vi "flyback scan with VIS monitor.vi"() -> ()   [LabVIEW 2015]
uses:
  <vilib>/DAQmx/read.llb/DAQmx Read (Analog 1D DBL 1Chan NSamp).vi
  <vilib>/DAQmx/write.llb/DAQmx Write (Digital 1D U32 1Chan NSamp).vi
  <vilib>/DAQmx/create/channels.llb/DAQmx Create Channel (DO-Digital Output).vi
  <vilib>/DAQmx/create/channels.llb/DAQmx Create Channel (CO-Pulse Generation-Time).vi
  <vilib>/DAQmx/configure/trigger.llb/DAQmx Start Trigger (Digital Edge).vi
  <vilib>/DAQmx/create/channels.llb/DAQmx Create Channel (AI-Voltage-Basic).vi
  <vilib>/DAQmx/configure/timing.llb/DAQmx Timing (Sample Clock).vi
  <vilib>/DAQmx/miscellaneous.llb/DAQmx Fill In Error Info.vi
  <vilib>/DAQmx/create/channels.llb/DAQmx Create Channel (CO-Pulse Generation-Frequency).vi
  <vilib>/DAQmx/configure/timing.llb/DAQmx Timing (Implicit).vi
  <resource>/objmgr/daqmx.rc
panel:
  out "current time(s)":i32
  in  "imaging time(s)":i32=40
  out "monitor signal":dbl[](graph)
  in  "path":path=path "C:/Users/Administrator/Desktop"
  out "monitor task":refnum<k21>
  out "CAM clock task":refnum<k21>
  in  "zero":dbl=30000.0 format="%#_13g"
  out "galvo task":refnum<k21>
  out "galvo clock task":refnum<k21>
  in  "aquire":bool
  out "current state":string
  in  "fps(Hz)":dbl=400.0 min=0.0 max=1000.0 step=1.0
  out "galvo x":dbl[](graph)
  out "galvo waveform":u32[](array[numeric])
  out "slope x":dbl=28768.0
  out "number of samples":u32
  out "point in t2":u32
  out "point in t1":u32
  in  "flyback time (ms)":dbl=1.09
  in  "exposure time (ms)":dbl=3.9
  out "retriggerable time(ms)":dbl=99.0
  in  "galvo clock rate":dbl=1000000.0 min=100000.0 max=1000000.0 format="%#_13g"
  in  "galvo scan amplitude":dbl=-0.56 min=-1.0 max=1.0
  in  "stop":bool
  # "exposure+flyback<=retriggerable"
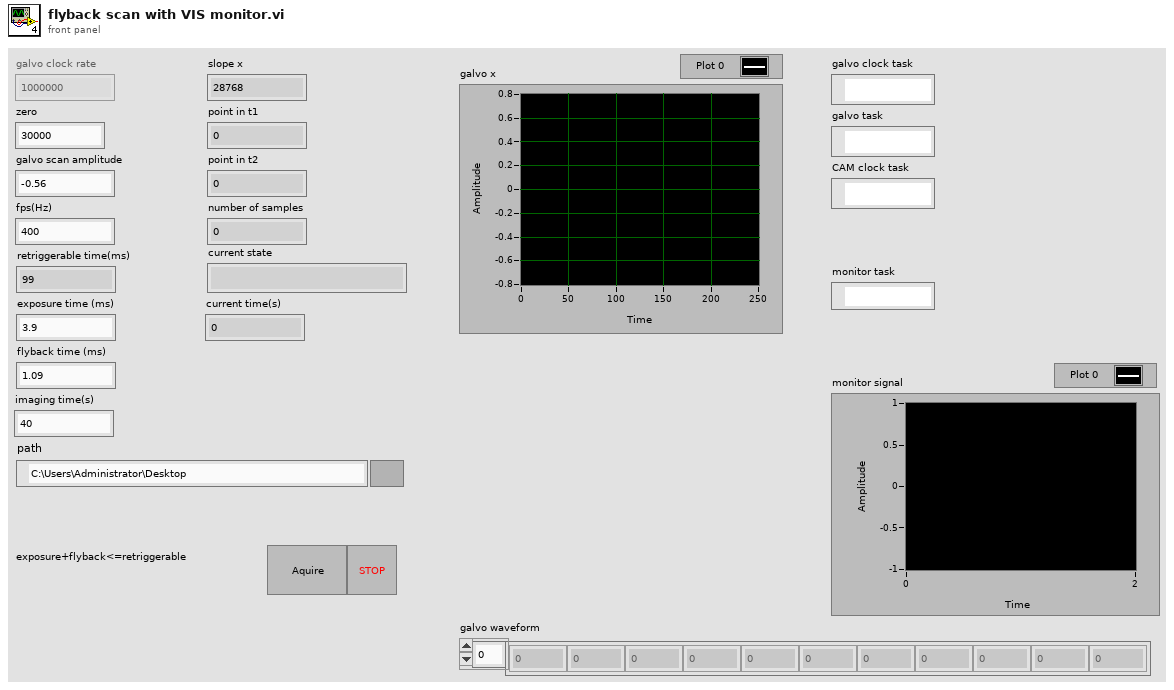
[diagram p1: front panel]
types:
  T1 = enum8{"Enabled", "Disabled", "Disabled and Grayed Out"}
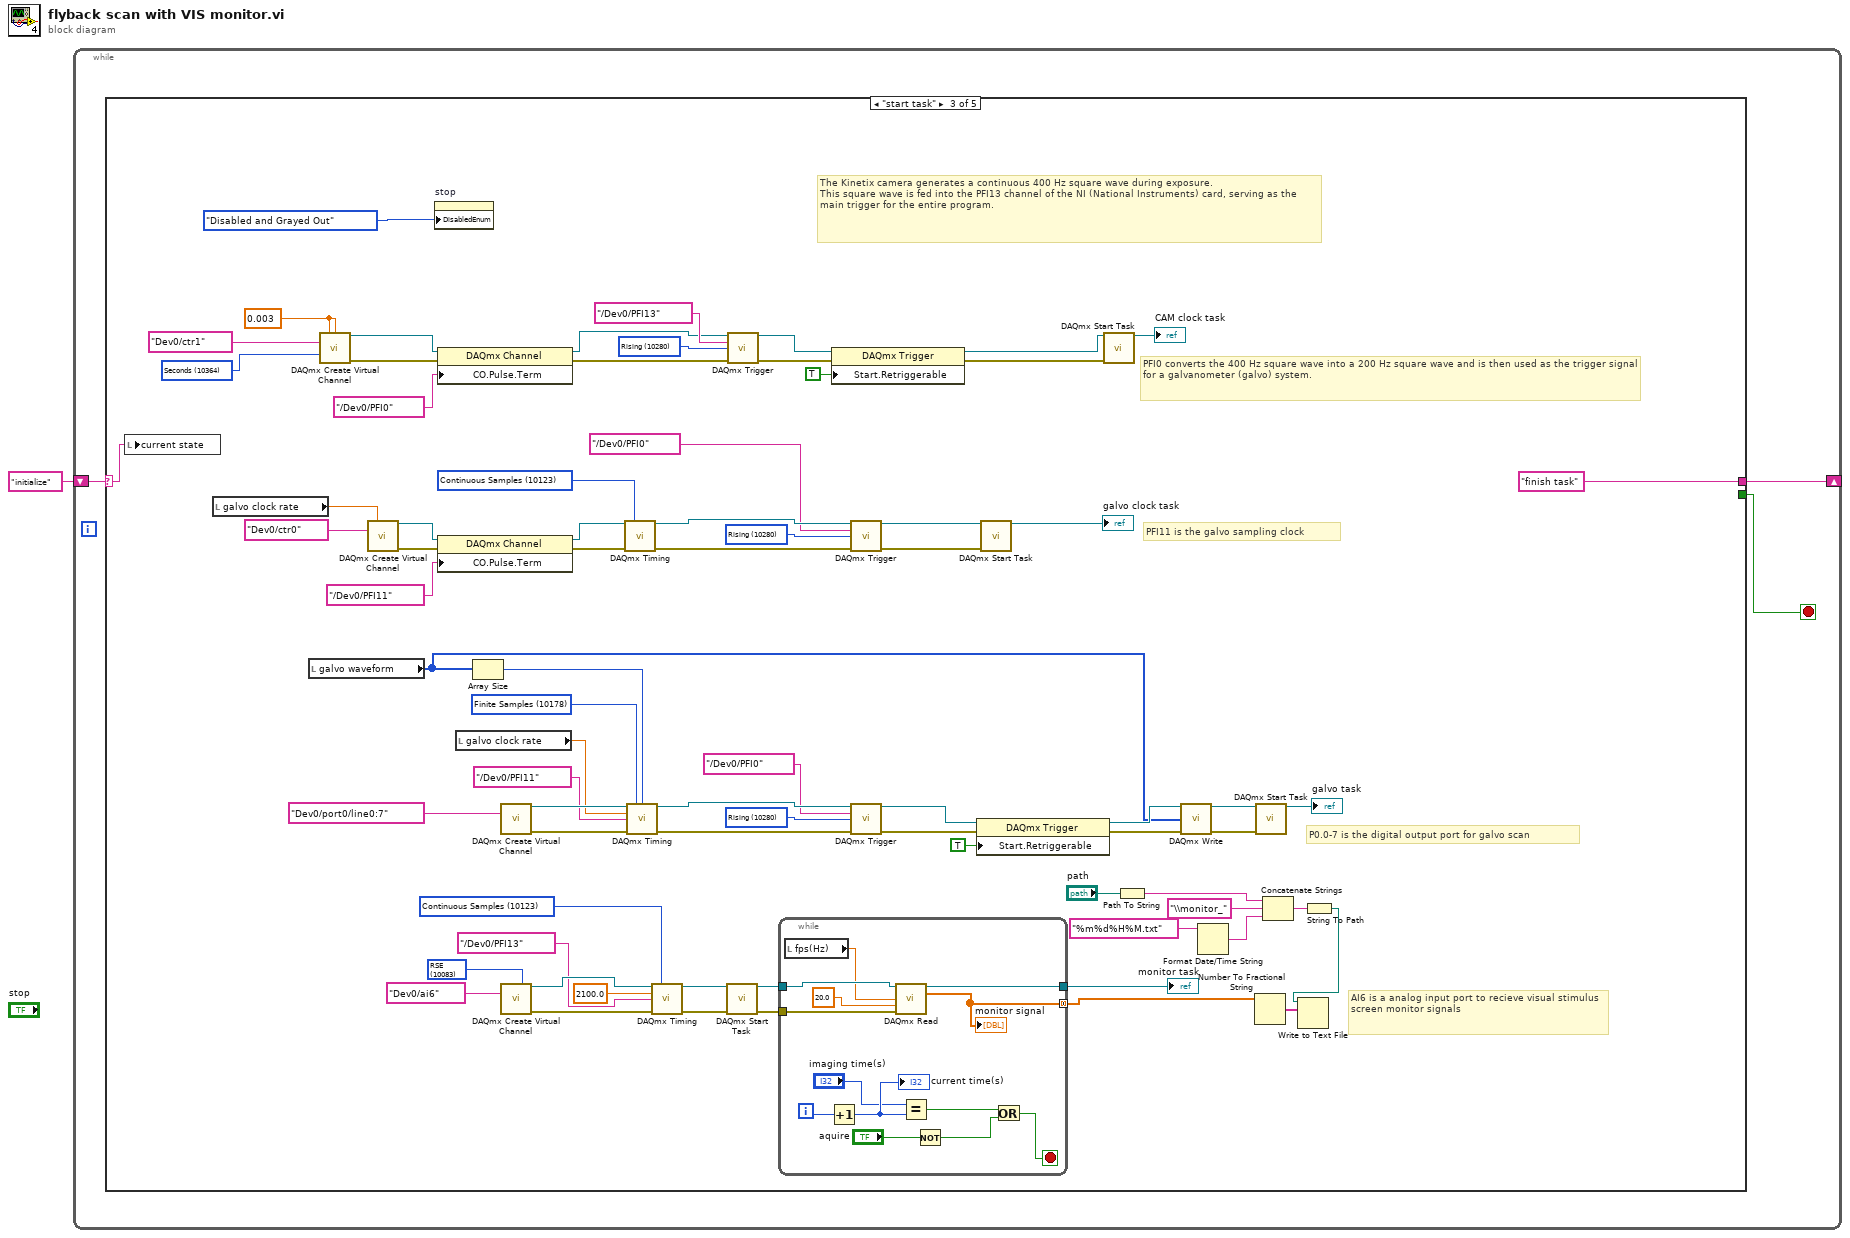
[diagram p0: block diagram]
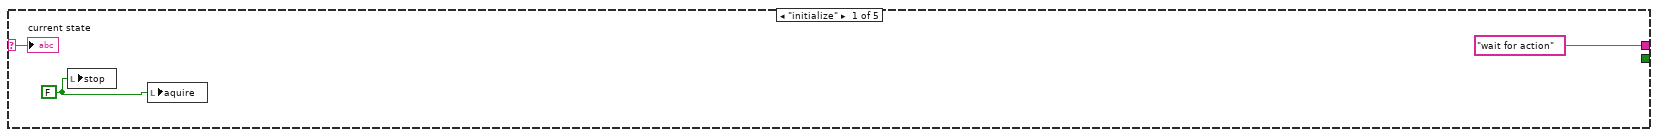
[diagram p2: hidden frame]
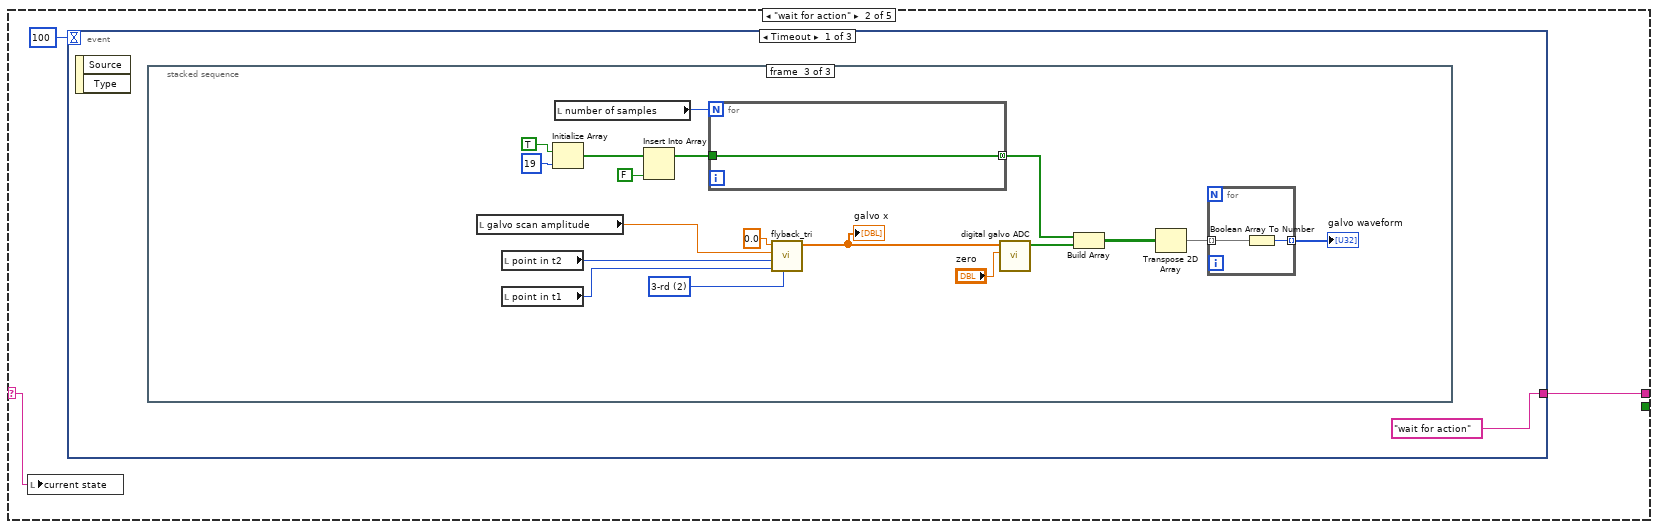
[diagram p3: hidden frame]
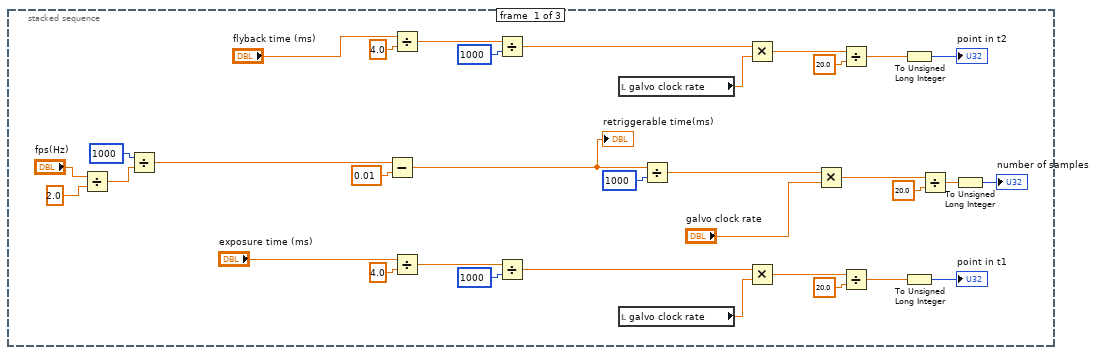
[diagram p4: hidden frame]
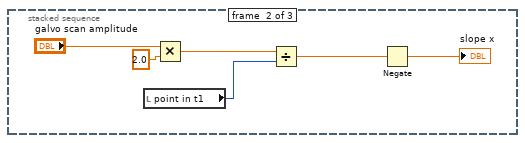
[diagram p5: hidden frame]
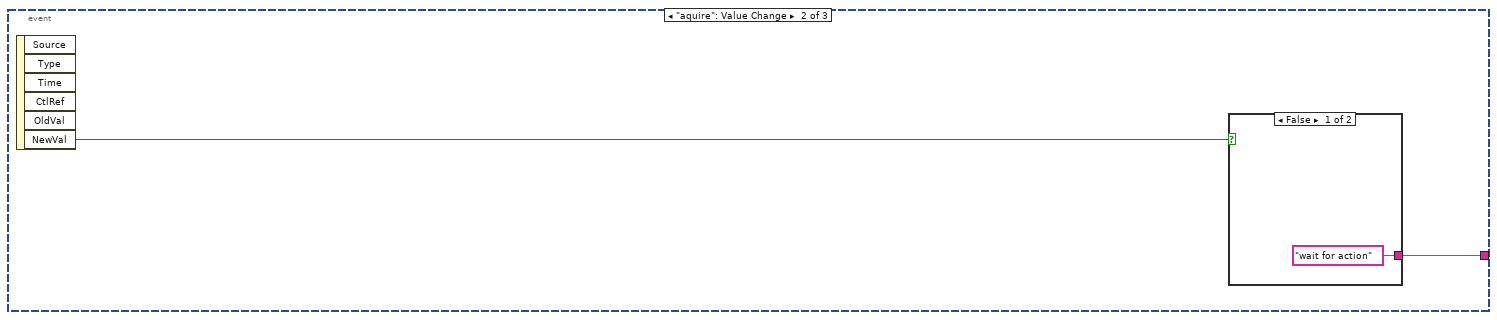
[diagram p6: hidden frame]
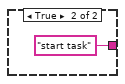
[diagram p7: hidden frame]
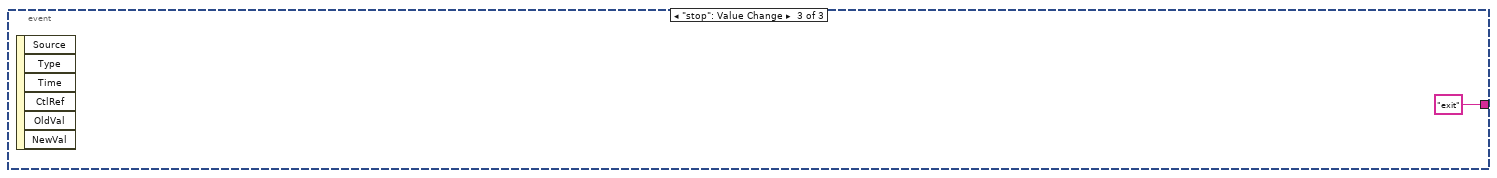
[diagram p8: hidden frame]
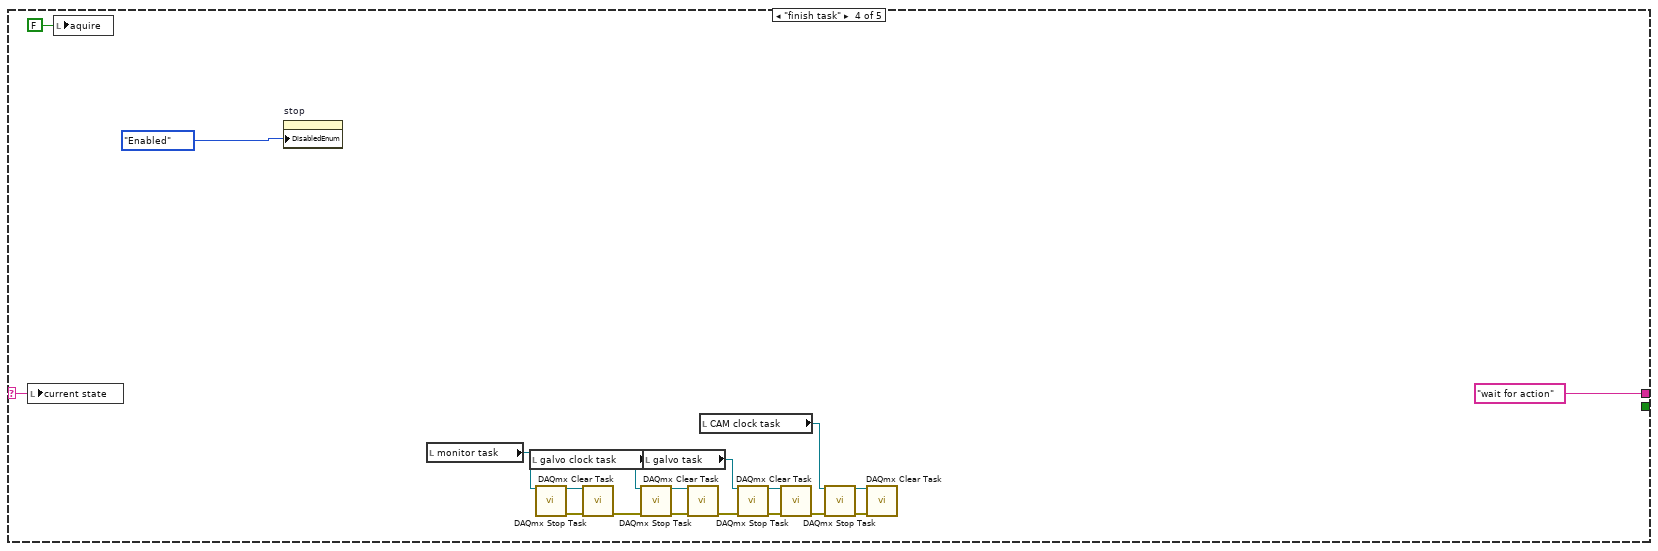
[diagram p9: hidden frame]
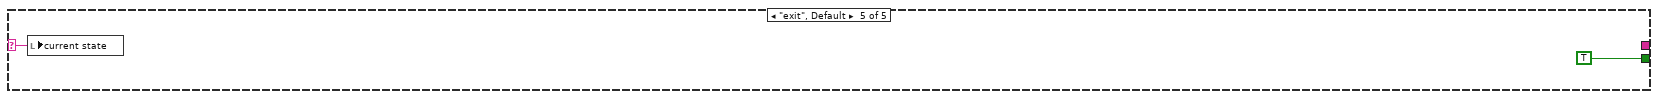
[diagram p10: hidden frame]
diagram:
  n1 = while {
    shift-right: [w3] -> _
    shift-left: "initialize" -> [w4]
    stop <- w2 stop-if-true
    n2 = case shown="\"start task\"" w4 {
      selector: w4 -> [w6 w8 w120 w184 w185]
      tunnel: ["wait for action" w9 "finish task" "wait for action" _] -> w3
      tunnel: [_ _ _ _ TRUE] -> w2
      frame "initialize" {
        w5 = FALSE ("stop")
        n3 = local write "stop"(w5) -> ()
        n4 = local write "aquire"(w5) -> ()
        "current state" <- w6
      }
      frame "wait for action" {
        n5 = local write "current state"(w8) -> ()
        n6 = event shown="[0] Timeout" {
          selector: _ -> [_ _ _]
          dyn-events: _ -> [_ _ _]
          timeout: 100 -> [_ _ _]
          tunnel: ["wait for action" w73 "exit"] -> w9
          event Timeout {
            n7 = event-data() -> ()  [unwired: 1 in, 2 out]
            n8 = stacked-sequence {
              frame #0 {
                n9 = Divide(x="fps(Hz)", y=2.0) -> (x/y=w12:dbl)
                n10 = Divide(x=1000 ("y"), y=w12) -> (x/y=w27:dbl)
                n11 = Subtract(x=w27, y=0.01) -> (x-y=w25:dbl)
                "retriggerable time(ms)" <- w25
                n12 = Divide(x="flyback time (ms)", y=4.0) -> (x/y=w16:dbl)
                n13 = Divide(x="exposure time (ms)", y=4.0) -> (x/y=w15:dbl)
                n14 = Divide(x=w16, y=1000) -> (x/y=w36:dbl)
                n15 = Divide(x=w15, y=1000) -> (x/y=w31:dbl)
                n16 = local read "galvo clock rate"() -> (w37:dbl)
                n17 = local read "galvo clock rate"() -> (w30:dbl)
                n18 = Divide(x=w25, y=1000) -> (x/y=w45:dbl)
                n19 = Multiply(x=w36, y=w37) -> (x*y=w35:dbl)
                n20 = Multiply(x=w31, y=w30) -> (x*y=w29:dbl)
                n21 = Multiply(x=w45, y="galvo clock rate") -> (x*y=w44:dbl)
                n22 = Divide(x=w35, y=20.0) -> (x/y=w22:dbl)
                n23 = Divide(x=w29, y=20.0) -> (x/y=w24:dbl)
                n24 = To Unsigned Long Integer(number=w22) -> (unsigned 32bit integer=→"point in t2":u32)
                n25 = To Unsigned Long Integer(number=w24) -> (unsigned 32bit integer=→"point in t1":u32)
                n26 = Divide(x=w44, y=20.0) -> (x/y=w42:dbl)
                n27 = To Unsigned Long Integer(number=w42) -> (unsigned 32bit integer=→"number of samples":u32)
              }
              frame #1 {
                n28 = local read "point in t1"() -> (w48:u32)
                n29 = Multiply(x="galvo scan amplitude", y=2.0) -> (x*y=w50:dbl)
                n30 = Divide(x=w50, y=w48) -> (x/y=w47:dbl)
                n31 = Negate(x=w47) -> (-x=→"slope x":dbl)
              }
              frame #2 {
                w52 = u16 2 items=["step", "line", "3-rd", "sine"] ("mode")
                n32 = local read "galvo scan amplitude"() -> (w55:dbl)
                n33 = local read "point in t2"() -> (w57:u32)
                n34 = local read "point in t1"() -> (w58:u32)
                n35 = Initialize Array(TRUE, 19 ("dimension size")) -> (w67:bool[])
                n36 = local read "number of samples"() -> (w59:u32)
                n37 = Insert Into Array(array=w67, new element=FALSE ("new element/subarray")) -> (w65:bool[])  [unwired: 1 in]
                n38 = for {
                  N: w59 -> [_]
                  tunnel: w65 -> [w72]
                  tunnel: [w72] -> w63 mode=concatenating
                }
                n39 = call "flyback_tri.vi"("mode"=w52, "points in t1"=w58, "points in t2"=w57, "p2"=w55, "p1"=0.0) -> ("array"=w53:dbl[])  [unwired: 6 in]
                "galvo x" <- w53
                n40 = call "digital galvo ADC.vi"("zero"="zero", "Analog waveform"=w53) -> ("Digital waveform"=w62:bool[])  [unwired: 9 in]
                n41 = Build Array(w63, w62) -> (w61:bool[][])
                n42 = Transpose 2D Array(2D array=w61) -> (transposed array=w64:bool[][])
                n43 = for {
                  tunnel: w64 -> [w70] mode=indexing
                  tunnel: [w71] -> w60 mode=indexing
                  n44 = Boolean Array To Number(Boolean array=w70) -> (number=w71:u32)
                }
                "galvo waveform" <- w60
              }
            }
          }
          event "aquire": Value Change {
            n45 = event-data() -> ("NewVal"=w74:bool)  [unwired: 1 in, 5 out]
            n46 = case shown="False" w74 {
              tunnel: ["wait for action" "start task"] -> w73
              frame False {
              }
              frame True {
              }
            }
          }
          event "stop": Value Change {
            n47 = event-data() -> ()  [unwired: 1 in, 6 out]
          }
        }
      }
      frame "start task" {
        w93 = 10123 items=["Finite Samples"=10178, "Continuous Samples"=10123, "Hardware Timed Single Point"=12522] ("sample mode")
        w98 = 10083 items=["Default"=-1, "RSE"=10083, "NRSE"=10078, "Differential"=10106, "Pseudodifferential"=12529] ("input terminal configuration")
        w102 = 10364 items=["Seconds"=10364] ("units")
        w103 = 0.003
        w114 = 10280 items=["Rising"=10280, "Falling"=10171] ("slope")
        w117 = 10280 items=["Rising"=10280, "Falling"=10171] ("edge")
        w127 = 10280 items=["Rising"=10280, "Falling"=10171] ("edge")
        w145 = 10178 items=["Finite Samples"=10178, "Continuous Samples"=10123, "Hardware Timed Single Point"=12522] ("sample mode")
        w144 = 10123 items=["Finite Samples"=10178, "Continuous Samples"=10123, "Hardware Timed Single Point"=12522] ("sample mode")
        # "AI6 is a analog input port to recieve visual stimulus screen monitor signals"
        # "P0.0-7 is the digital output port for galvo scan"
        # "PFI11 is the galvo sampling clock"
        # "PFI0 converts the 400 Hz square wave into a 200 Hz square wave and is then used as the trigger signal for a galvanometer (galvo) system."
        # "The Kinetix camera generates a continuous 400 Hz square wave during exposure. \nThis square wave is fed into the PFI13 channel of the NI (National Instruments) card, serving as the main trigger for the entire program."
        n48 = local write "current state"(w120) -> ()
        n49 = local read "galvo clock rate"() -> (w115:dbl)
        n50 = local read "galvo waveform"() -> (w135:u32[])
        n51 = call-poly <vilib>:"DAQmx Create Virtual Channel.vi"("high time"=w103, "low time"=w103, "counter"=tag "Dev0/ctr1", "units"=w102) -> ("task out"=w107:refnum<k21>, "error out"=w106:errorcluster)  [unwired: 10 in]
        n52 = call-poly <vilib>:"DAQmx Create Virtual Channel.vi"("frequency"=w115, "counter"=tag "Dev0/ctr0") -> ("task out"=w124:refnum<k21>, "error out"=w123:errorcluster)  [unwired: 12 in]
        n53 = property on="stop" class="Bool (strict)"("DisabledEnum"=T1."Disabled and Grayed Out" ("Disabled")) -> ()  [unwired: 2 in, 2 out]
        n54 = property class="DAQmx Channel"(reference=w107, error in=w106, "CO.Pulse.Term"=tag "/Dev0/PFI0") -> (reference out=w101:refnum<k21>, error out=w100:errorcluster)
        n55 = property class="DAQmx Channel"(reference=w124, error in=w123, "CO.Pulse.Term"=tag "/Dev0/PFI11") -> (reference out=w122:refnum<k21>, error out=w121:errorcluster)
        n56 = local read "galvo clock rate"() -> (w132:dbl)
        n57 = Array Size(array=w135) -> (size(s)=w134:i32)
        n58 = call-poly <vilib>:"DAQmx Create Virtual Channel.vi"("lines"=tag "Dev0/port0/line0:7") -> ("task out"=w138:refnum<k21>, "error out"=w139:errorcluster)  [unwired: 13 in]
        n59 = call-poly <vilib>:"DAQmx Create Virtual Channel.vi"("input terminal configuration"=w98, "physical channels"=tag "Dev0/ai6") -> ("task out"=w97:refnum<k21>, "error out"=w94:errorcluster)  [unwired: 12 in]
        n60 = call-poly <vilib>:"DAQmx Timing.vi"("task/channels in"=w122, "sample mode"=w144, "error in"=w121) -> ("task out"=w128:refnum<k21>, "error out"=w129:errorcluster)  [unwired: 11 in]
        n61 = call-poly <vilib>:"DAQmx Timing.vi"("task/channels in"=w138, "sample mode"=w145, "samples per channel"=w134, "rate"=w132, "source"=tag "/Dev0/PFI11" ("Sample Clock Source"), "error in"=w139) -> ("task out"=w149:refnum<k21>, "error out"=w150:errorcluster)  [unwired: 8 in]
        n62 = call-poly <vilib>:"DAQmx Timing.vi"("task/channels in"=w97, "sample mode"=w93, "rate"=2100.0, "source"=tag "/Dev0/PFI13", "error in"=w94) -> ("task out"=w96:refnum<k21>, "error out"=w95:errorcluster)  [unwired: 9 in]
        n63 = call <vilib>:"DAQmx Start Task.vi"("task/channels in"=w96, "error in"=w95) -> ("task out"=w90:refnum<k21>, "error out"=w89:errorcluster)  [unwired: 12 in]
        n64 = call-poly <vilib>:"DAQmx Trigger.vi"("task/channels in"=w101, "source"=tag "/Dev0/PFI13" ("source of ticks"), "edge"=w117, "error in"=w100) -> ("task out"=w118:refnum<k21>, "error out"=w112:errorcluster)  [unwired: 10 in]
        n65 = while {
          tunnel: w89 -> [w164]
          tunnel: [w162] -> w81 mode=concatenating
          tunnel: w90 -> [w165]
          tunnel: [w163] -> w88
          i -> [w154]
          stop <- w155 stop-if-true
          n66 = local read "fps(Hz)"() -> (w153:dbl)
          n67 = Increment(x=w154) -> (x+1=w159:i32)
          "current time(s)" <- w159
          n68 = call-poly <vilib>:"DAQmx Read.vi"("task/channels in"=w165, "number of samples per channel"=w153, "timeout"=20.0, "error in"=w164) -> ("task out"=w163:refnum<k21>, "data"=w162:dbl[])  [unwired: 9 in, 1 out]
          "monitor signal" <- w162
          n69 = Equal?(x="imaging time(s)", y=w159) -> (x = y?=w157:bool)
          n70 = Not(x="aquire") -> (.not. x?=w158:bool)
          n71 = Or(x=w157, y=w158) -> (x .or. y?=w155:bool)
        }
        "monitor task" <- w88
        n72 = property class="DAQmx Trigger"(reference=w118, error in=w112, "Start.Retriggerable"=TRUE) -> (reference out=w110:refnum<k21>, error out=w109:errorcluster)
        n73 = call-poly <vilib>:"DAQmx Trigger.vi"("task/channels in"=w128, "source"=tag "/Dev0/PFI0", "edge"=w127, "error in"=w129) -> ("task out"=w131:refnum<k21>, "error out"=w130:errorcluster)  [unwired: 10 in]
        n74 = call-poly <vilib>:"DAQmx Trigger.vi"("task/channels in"=w149, "source"=tag "/Dev0/PFI0", "edge"=w114, "error in"=w150) -> ("task out"=w147:refnum<k21>, "error out"=w146:errorcluster)  [unwired: 10 in]
        n75 = property class="DAQmx Trigger"(reference=w147, error in=w146, "Start.Retriggerable"=TRUE) -> (reference out=w151:refnum<k21>, error out=w152:errorcluster)
        n76 = call <vilib>:"DAQmx Start Task.vi"("task/channels in"=w131, "error in"=w130) -> ("task out"=→"galvo clock task":refnum<k21>)  [unwired: 12 in, 1 out]
        n77 = call <vilib>:"DAQmx Start Task.vi"("task/channels in"=w110, "error in"=w109) -> ("task out"=→"CAM clock task":refnum<k21>)  [unwired: 12 in, 1 out]
        n78 = Path To String(path="path") -> (string=w83:string)
        n79 = call-poly <vilib>:"DAQmx Write.vi"("task/channels in"=w151, "data"=w135, "error in"=w152) -> ("task out"=w140:refnum<k21>, "error out"=w141:errorcluster)  [unwired: 10 in, 1 out]
        n80 = Format Date/Time String(time format string (%c)="%m%d%H%M.txt") -> (date/time string=w87:string)  [unwired: 2 in]
        n81 = Number To Fractional String(number=w81) -> (F-format string=w82:string[])  [unwired: 3 in]
        n82 = call <vilib>:"DAQmx Start Task.vi"("task/channels in"=w140, "error in"=w141) -> ("task out"=→"galvo task":refnum<k21>)  [unwired: 12 in, 1 out]
        n83 = Concatenate Strings(w83, "\\monitor_", w87) -> (w85:string)
        n84 = String To Path(string=w85) -> (path=w79:path)
        n85 = Write to Text File(file (use dialog)=w79, text=w82) -> ()  [unwired: 2 in, 3 out]
      }
      frame "finish task" {
        n86 = local write "current state"(w184) -> ()
        n87 = local write "aquire"(FALSE ("aquire")) -> ()
        n88 = property on="stop" class="Bool (strict)"("DisabledEnum"=T1."Enabled" ("Disabled")) -> ()  [unwired: 2 in, 2 out]
        n89 = local read "monitor task"() -> (w171:refnum<k21>)
        n90 = local read "galvo clock task"() -> (w180:refnum<k21>)
        n91 = call <vilib>:"DAQmx Stop Task.vi"("task/channels in"=w171) -> ("task out"=w170:refnum<k21>, "error out"=w172:errorcluster)  [unwired: 13 in]
        n92 = call <vilib>:"DAQmx Clear Task.vi"("task in"=w170, "error in"=w172) -> ("error out"=w167:errorcluster)  [unwired: 13 in]
        n93 = call <vilib>:"DAQmx Stop Task.vi"("task/channels in"=w180, "error in"=w167) -> ("task out"=w181:refnum<k21>, "error out"=w179:errorcluster)  [unwired: 12 in]
        n94 = local read "galvo task"() -> (w174:refnum<k21>)
        n95 = call <vilib>:"DAQmx Clear Task.vi"("task in"=w181, "error in"=w179) -> ("error out"=w169:errorcluster)  [unwired: 13 in]
        n96 = local read "CAM clock task"() -> (w173:refnum<k21>)
        n97 = call <vilib>:"DAQmx Stop Task.vi"("task/channels in"=w174, "error in"=w169) -> ("task out"=w177:refnum<k21>, "error out"=w176:errorcluster)  [unwired: 12 in]
        n98 = call <vilib>:"DAQmx Clear Task.vi"("task in"=w177, "error in"=w176) -> ("error out"=w168:errorcluster)  [unwired: 13 in]
        n99 = call <vilib>:"DAQmx Stop Task.vi"("task/channels in"=w173, "error in"=w168) -> ("task out"=w178:refnum<k21>, "error out"=w175:errorcluster)  [unwired: 12 in]
        n100 = call <vilib>:"DAQmx Clear Task.vi"("task in"=w178, "error in"=w175) -> ()  [unwired: 13 in, 1 out]
      }
      frame "exit", Default {
        n101 = local write "current state"(w185) -> ()
      }
    }
  }
